vi "Prepare Data for Review.vi"(10 "PI pos (um)":dbl[](array[numeric]), 11 "Timestamps (ms)":u64[](array[numeric])) -> (0 "total frames":i32, 1 "PI pos (um) out":dbl[](array[numeric]), 2 "dts":u64[](array[numeric]), 3 "Time (s)":dbl[](array[numeric]), 5 "PIFOC Graph":cluster{dbl[], "PI pos (um)":dbl[]})   [LabVIEW 2020]
uses:
  _Globals/Global Controls.vi
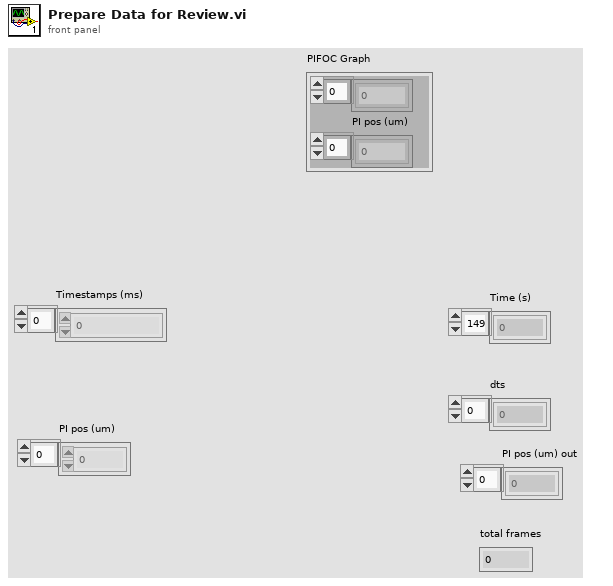
[diagram p1: front panel]
types:
  T1 = typedef "Review Ctrl Refs.ctl" = cluster{"RevFrame":refnum<vi>, "dts (ms)":refnum<vi>, "PIFOC Positions":refnum<vi>}
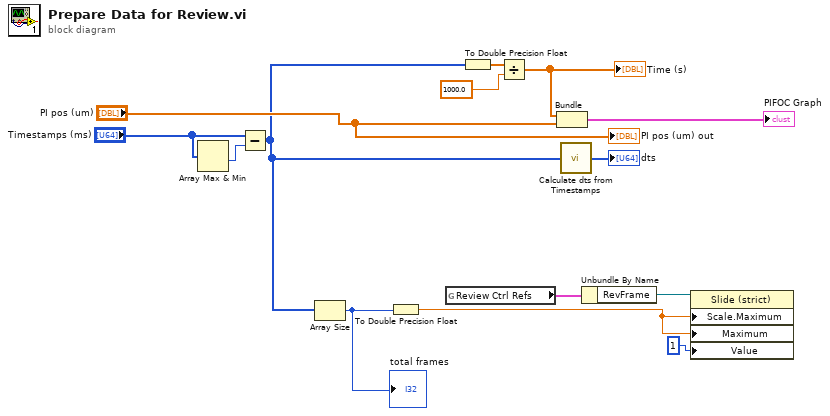
[diagram p0: block diagram]
diagram:
  n1 = Array Max & Min(array="Timestamps (ms)") -> (min value=w6:u64)  [unwired: 3 out]
  n2 = Subtract(x="Timestamps (ms)", y=w6) -> (x-y=w5:u64[])
  n3 = Array Size(array=w5) -> (size(s)=w9:i32)
  "total frames" <- w9
  n4 = To Double Precision Float(number=w9) -> (double precision float=w13:dbl)
  n5 = global read "Global Controls.vi" "Review Ctrl Refs"() -> (w11:T1)
  n6 = To Double Precision Float(number=w5) -> (double precision float=w3:dbl[])
  n7 = Divide(x=w3, y=1000.0) -> (x/y=w2:dbl[])
  "Time (s)" <- w2
  n8 = Bundle(w2, "PI pos (um)"="PI pos (um)") -> (→"PIFOC Graph":cluster{dbl[], "PI pos (um)":dbl[]})  [unwired: 1 in]
  n9 = call "Calculate dts from Timestamps.vi"("TimeStamps"=w5) -> ("dts"=→"dts":u64[])  [unwired: 4 in]
  n10 = Unbundle By Name(w11) -> ("RevFrame"=w12:refnum<vi>)
  n11 = property class="Slide (strict)"(reference=w12, "Scale.Maximum"=w13, "Maximum"=w13, "Value"=1 ("RevFrame")) -> ()  [unwired: 1 in, 2 out]
  "PI pos (um) out" <- "PI pos (um)"
